vi "last_dust_event_query.vi"(8 "error in (no error)":errorcluster, 11 "Small?":bool) -> (0 "error out":errorcluster, 3 "id_dust_event":i64)   [LabVIEW 2015]
uses:
  <vilib>/addons/database/_DB Variant To Data/Database Variant To Data.xnode
panel:
  out "SQL Query":string="SELECT\n  max(id_dust_event)\nFROM\n   dust_event;"
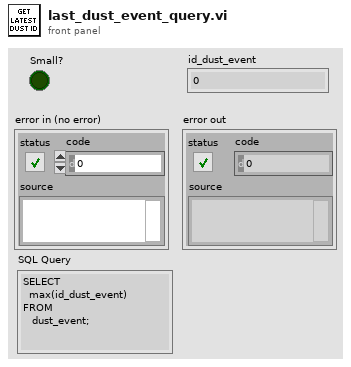
[diagram p1: front panel]
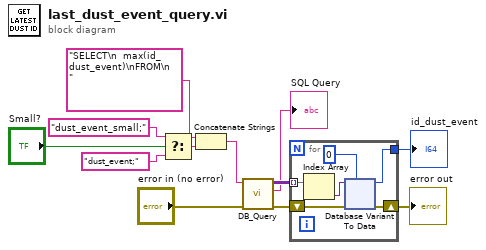
[diagram p0: block diagram]
diagram:
  n1 = Select(t="dust_event_small;" ("SQL query"), s="Small?", f="dust_event;" ("SQL query")) -> (s? t:f=w3:string)
  n2 = Concatenate Strings("SELECT\n  max(id_dust_event)\nFROM\n   " ("SQL query"), w3) -> (w1:string)
  n3 = call "DB_Query.vi"("error in (no error)"="error in (no error)", "Parameterized Query"=w1) -> ("error out"=w9:errorcluster, "Query in Standard Format"=→"SQL Query":string, "Results"=w8:variant[][])  [unwired: 7 in]
  n4 = for {
    tunnel: [w16] -> w12
    tunnel: w8 -> [w14] mode=indexing
    shift-right: [w13] -> w6
    shift-left: w9 -> [w15]
    n5 = Index Array(array=w14) -> (element=w18:variant)  [unwired: 1 in]
    n6 = xnode "Database Variant To Data"("database variant"=w18, "error in (no error)"=w15, "type"=i64 0) -> ("data"=w16:i64, "error out"=w13:errorcluster)
  }
  "id_dust_event" <- w12
  "error out" <- w6
